vi "sub_ForceTime.vi"(8 "error in":errorcluster) -> (0 "error out":errorcluster, 3 "Force wf_T":waveform(dbl)(graph))   [LabVIEW 2016]
uses:
  ctl/Data_buf_cmd.ctl
  <vilib>/Waveform/WDTOps.llb/WDT Append Waveforms DBL.vi
panel:
  out "Bonding only graph":waveform(dbl)(graph)
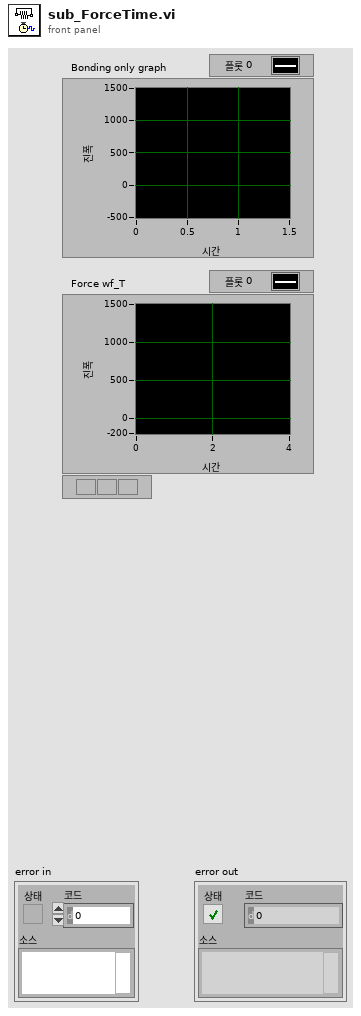
[diagram p1: front panel]
types:
  T1 = typedef "UI_ctl.ctl" = cluster{"Heater temp":refnum<vi>, "Heater chart":refnum<vi>, "vacuum (kpa)":refnum<vi>, "Balance xy graph":refnum<vi>, "Strain chart w cal":refnum<vi>, "Pickup force":refnum<vi>, "Pickup time":refnum<vi>, "Force chart":refnum<vi>, "Force graph T":refnum<vi>, "vacuum chart":refnum<vi>, "vacuum rt":refnum<vi>, "Strain raw graph":refnum<vi>, "Strain raw chart":refnum<vi>, "Bonding time":refnum<vi>, "Bonding force":refnum<vi>, "Balance":refnum<vi>, "Filtered force graph":refnum<vi>, "ROI intensity":refnum<vi>, "Heater_rt":refnum<vi>, "Detach force":refnum<vi>, "Force rt":refnum<vi>, "Mixed signal":refnum<vi>}
  T2 = typedef "Data_buf_cmd.ctl" = enum16{"insert", "default", "create", "clear"}
  T3 = typedef "config_ctl.ctl" = cluster{"Lower Cut-Off":dbl, "Vacuum Trigger level":dbl, "state settings":cluster{"method":enum32{"histogram", "peak", "auto select"}, "histogram size":i32, "histogram method":enum16{"mode"}, "reserved":dbl}, "SPA-300 Setting":cluster{"Bonding force (g)":dbl, "Bonding time (ms)":dbl, "Pickup force (g)":dbl, "Pickup time (ms)":dbl, "Speed":enum16{"Slow", "Fast"}}, "sensor file":path}
  T4 = cluster{"falling_index":dbl, "rising_index":dbl, "falling_t":dbl, "rising_t":dbl}
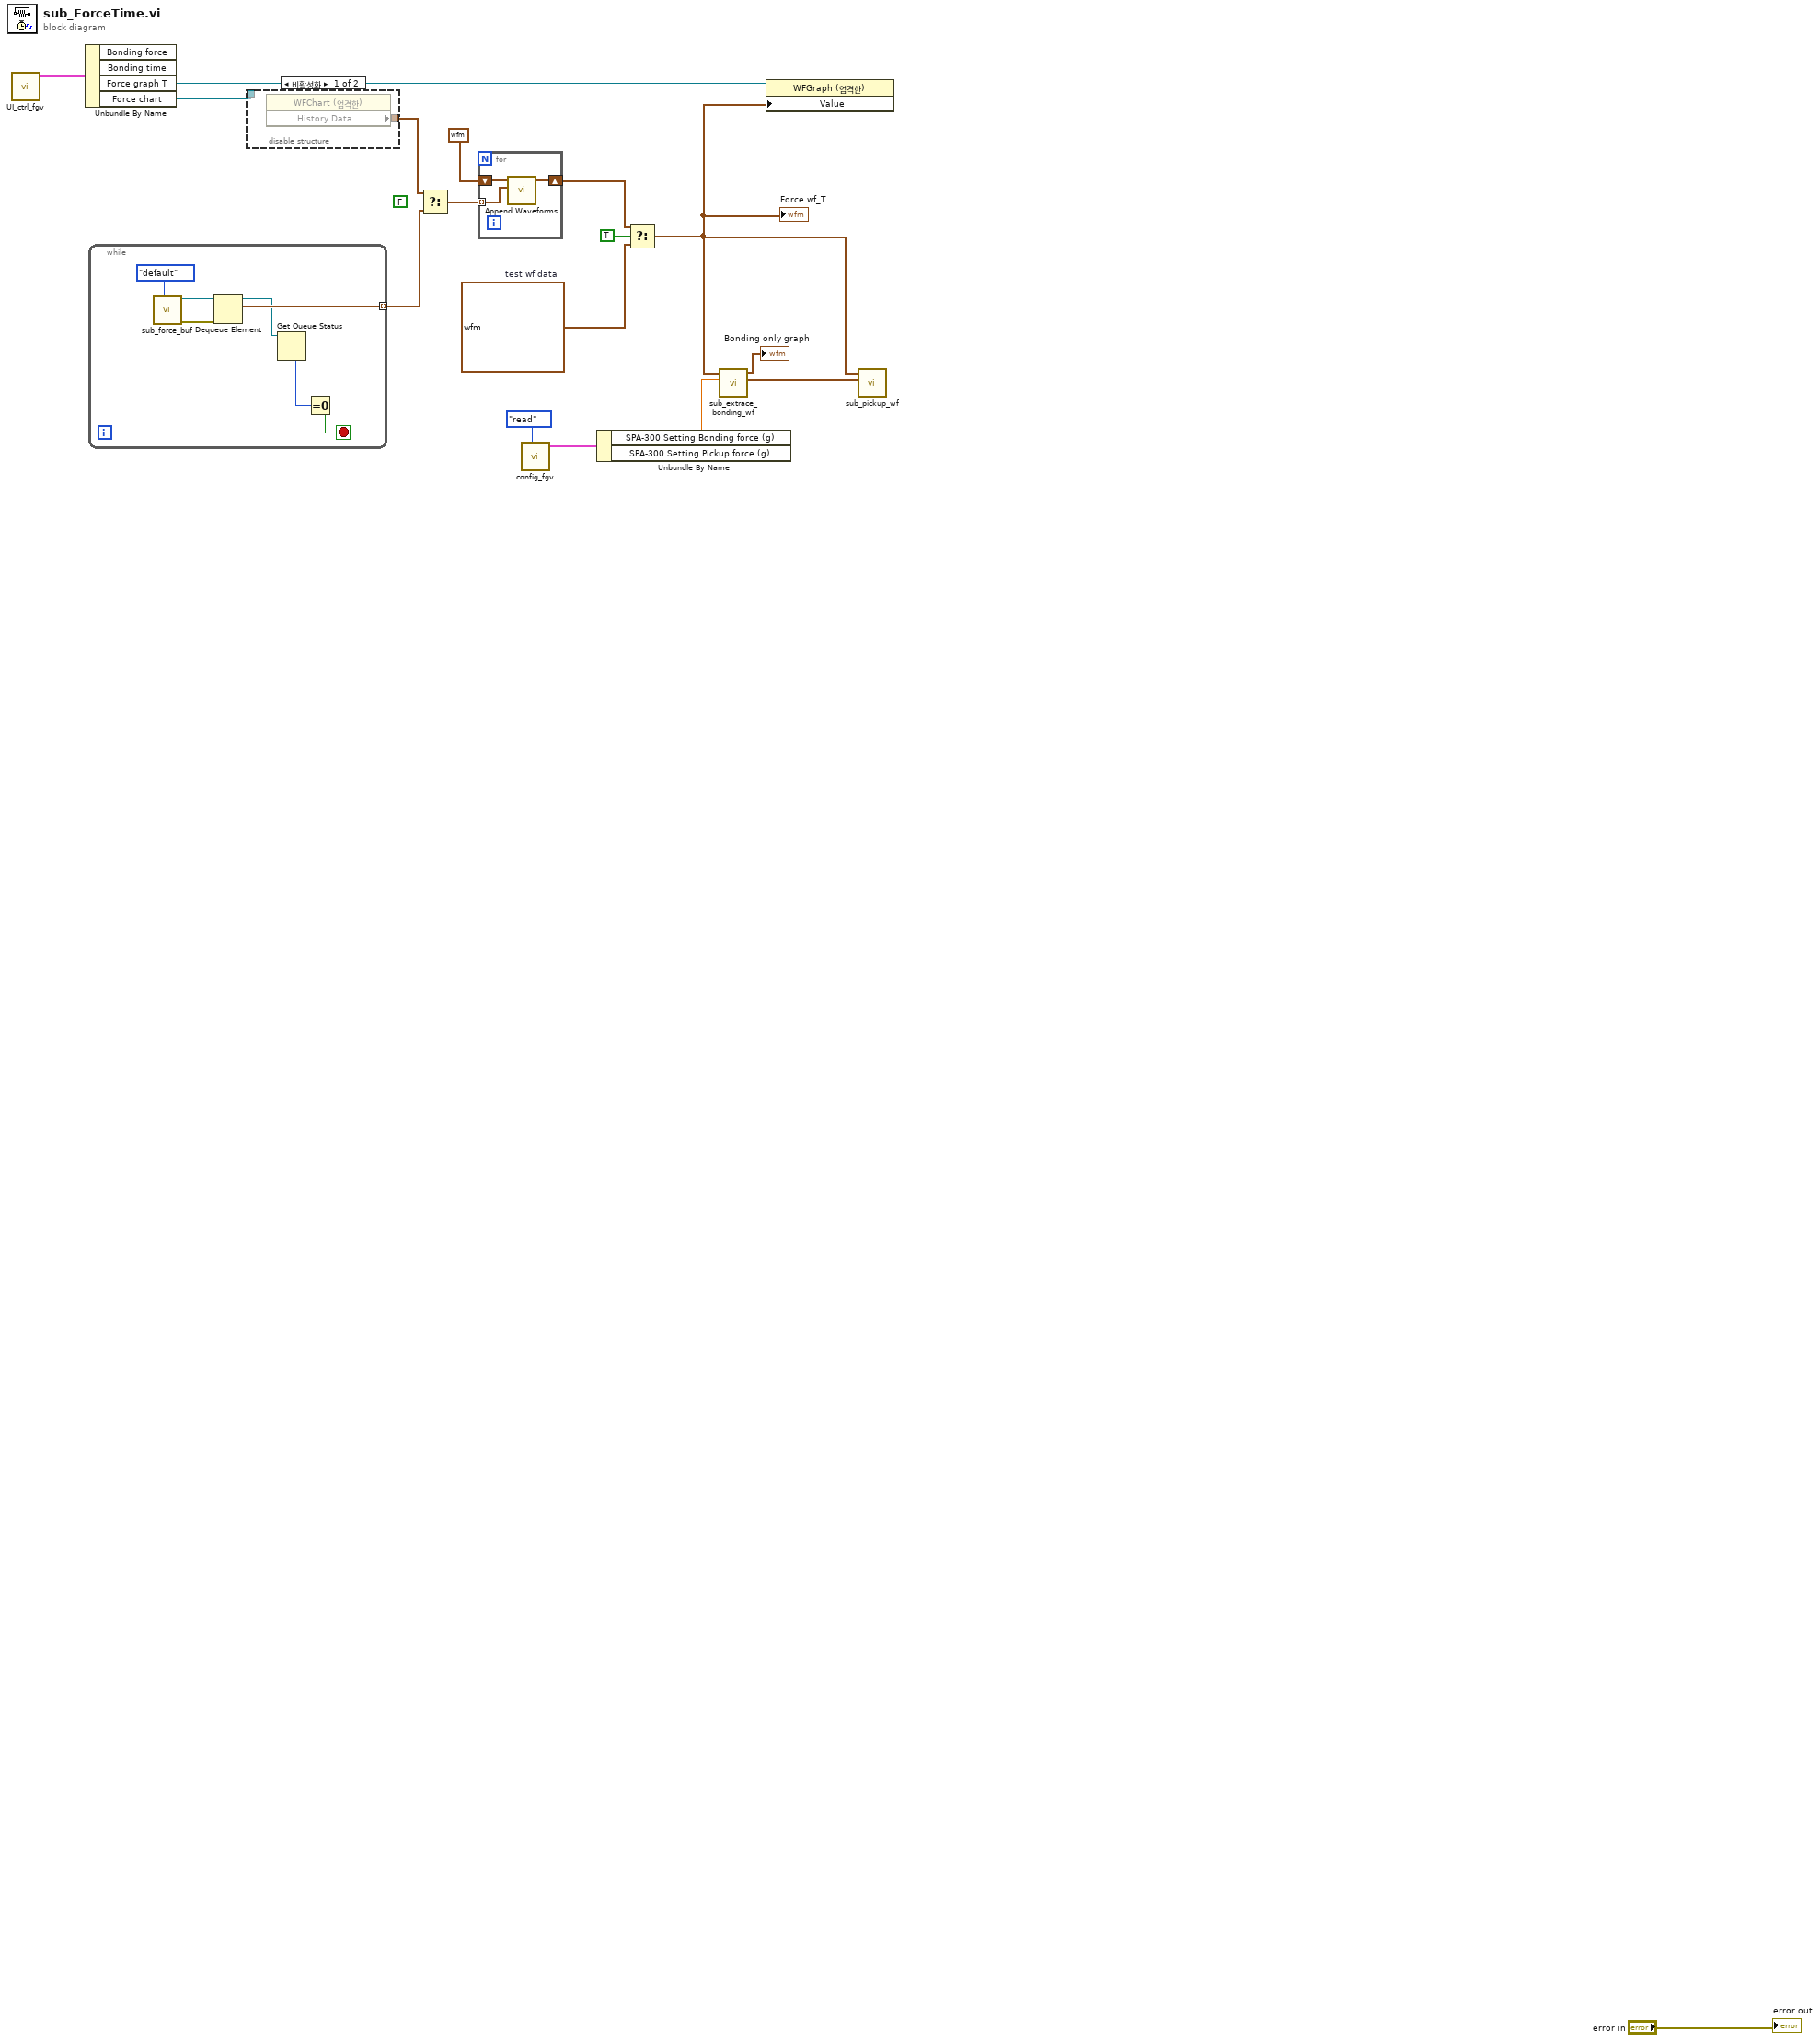
[diagram p0: block diagram]
diagram:
  w10 = waveform(dbl) {"t0"=timestamp(0 s since 1904-01-01), "dt"=0.00024, "Y"=array[12800 elements]}  # test wf data
  n1 = call "UI_ctrl_fgv.vi"() -> ("UI cluster out"=w18:T1)  [unwired: 11 in]
  n2 = Unbundle By Name(w18) -> ("Force graph T"=w13:refnum<vi>, "Force chart"=w15:refnum<vi>)  [unwired: 2 out]
  n3 = while {
    tunnel: [w23] -> w1 mode=indexing
    stop <- w21 stop-if-true
    n4 = call "sub_force_buf.vi"("cmd"=Data_buf_cmd."default") -> ("error out"=w24:errorcluster, "queue out"=w25:refnum<queue>)  [unwired: 9 in]
    n5 = Dequeue Element(queue=w25, error in (no error)=w24) -> (queue out=w22:refnum<queue>, element=w23:waveform(dbl))  [unwired: 1 in, 2 out]
    n6 = Get Queue Status(queue=w22) -> (# elements in queue=w20:i32)  [unwired: 2 in, 7 out]
    n7 = Equal To 0?(x=w20) -> (x = 0?=w21:bool)
  }
  n8 = disable-structure shown="비활성화" {
    disable-tunnel: w15 -> [w27 _]
    disable-tunnel: [w26 _] -> w2
    frame Disabled {
      n9 = property class="WFChart (엄격한)"(reference=w27) -> ("History Data"=w26:waveform(dbl)[])  [unwired: 1 in, 2 out]
    }
    frame Enabled {
    }
  }
  n10 = Select(t=w2, s=FALSE, f=w1) -> (s? t:f=w3:waveform(dbl)[])
  n11 = for {
    shift-right: [w28] -> w12
    shift-left: waveform(dbl) {"t0"=timestamp(0 s since 1904-01-01), "dt"=0.00024, "Y"=[]} -> [w30]
    tunnel: w3 -> [w29] mode=indexing
    n12 = call-poly <vilib>:"Append Waveforms.vi"("waveform B"=w29, "waveform A"=w30) -> ("waveform out"=w28:waveform(dbl))  [unwired: 8 in, 1 out]
  }
  n13 = call "config_fgv.vi"("cmd"=enum16{"write", "read", "ini"}."read") -> ("Config out"=w17:T3)  [unwired: 9 in, 1 out]
  n14 = Unbundle By Name(w17) -> ("SPA-300 Setting.Bonding force (g)"=w9:dbl)  [unwired: 1 out]
  n15 = Select(t=w12, s=TRUE, f=w10) -> (s? t:f=w5:waveform(dbl))
  "Force wf_T" <- w5
  n16 = call "sub_extrace_bonding_wf.vi"("Bonding force"=w9, "Trigger graph"=w5) -> ("b_info"=w6:T4, "Bonding"=→"Bonding only graph":waveform(dbl))  [unwired: 8 in]
  n17 = property class="WFGraph (엄격한)"(reference=w13, "Value"=w5) -> ()  [unwired: 1 in, 2 out]
  n18 = call "sub_pickup_wf.vi"("b_info"=w6, "wf"=w5) -> ()  [unwired: 9 in, 1 out]
  "error out" <- "error in"
